vi "Set Gate Function.vi"(6 "EF":u32(ring) items=["Normal"=0, "EF_OR"=1048576, "EF_AND"=2097152, "EF_XOR"=3145728], 8 "error in (no error)":errorcluster, 9 "CD":u32(ring) items=["Normal"=0, "CD_OR"=262144, "CD_AND"=524288, "CD_XOR"=786432], 10 "AB":u32(ring) items=["Normal"=0, "AB_OR"=65536, "AB_AND"=131072, "AB_XOR"=196608], 11 "DG Number":i32) -> (0 "error out":errorcluster)   [LabVIEW 2009]
doc: "long Set_ClockParameters(BOOL ClockEnable, unsigned long DivideBy, unsigned long ClockSource, long DG_Number);"
uses:
  BME DLL/DelayGenerator.dll
panel:
  out "Result":u32 format="%08x"
  # "NOTICE -- YOU MUST LEAVE THIS NOTICE IN PLACE.  PER THE TERMS OF THE LICENSE BELOW, YOU MAY SUBLICENSE THIS SOFTWARE \nIN ANY WAY THAT DOES NOT CONFLICT WITH THIS LICENSE.\n\n### BSD License (http://www.opensource.org/licenses/bsd-license.php) Begin ###\n \nCopyright (c) 2011, Applied Energetics, http://www.appliedenergetics.com,\n                               Richard Schwerdtfeger, <rschwerdtfeger@appliedenergetics.com>\n\nAll rights reserved.\n\nRedistribution and use in source and binary forms, with or without modification, are permitted provided that the \nfollowing conditions are met:\n\n    * Redistributions of source code must retain the above copyright notice, this list of conditions and the following disclaimer.\n    * Redistributions in binary form must reproduce the above copyright notice, this list of conditions and the following disclaimer \n       in the documentation and/or other materials provided with the distribution.\n    * Neither the name of Richard Schwerdtfeger, Applied Energetics, Inc., nor the names of its contributors may be used to \n       endorse or promote products derived from this software without specific prior written permission.\n\nTHIS SOFTWARE IS PROVIDED BY THE COPYRIGHT HOLDERS AND CONTRIBUTORS \"AS IS\" AND ANY EXPRESS OR IMPLIED WARRANTIES, \nINCLUDING, BUT NOT LIMITED TO, THE IMPLIED WARRANTIES OF MERCHANTABILITY AND FITNESS FOR A PARTICULAR PURPOSE ARE \nDISCLAIMED. IN NO EVENT SHALL THE COPYRIGHT OWNER OR CONTRIBUTORS BE LIABLE FOR ANY DIRECT, INDIRECT, INCIDENTAL,\n SPECIAL, EXEMPLARY, OR CONSEQUENTIAL DAMAGES (INCLUDING, BUT NOT LIMITED TO, PROCUREMENT OF SUBSTITUTE GOODS OR \nSERVICES; LOSS OF USE, DATA, OR PROFITS; OR BUSINESS INTERRUPTION) HOWEVER CAUSED AND ON ANY THEORY OF LIABILITY, \nWHETHER IN CONTRACT, STRICT LIABILITY, OR TORT (INCLUDING NEGLIGENCE OR OTHERWISE) ARISING IN ANY WAY OUT OF THE USE \nOF THIS SOFTWARE, EVEN IF ADVISED OF THE POSSIBILITY OF SUCH DAMAGE.\n\n### BSD License End ###"
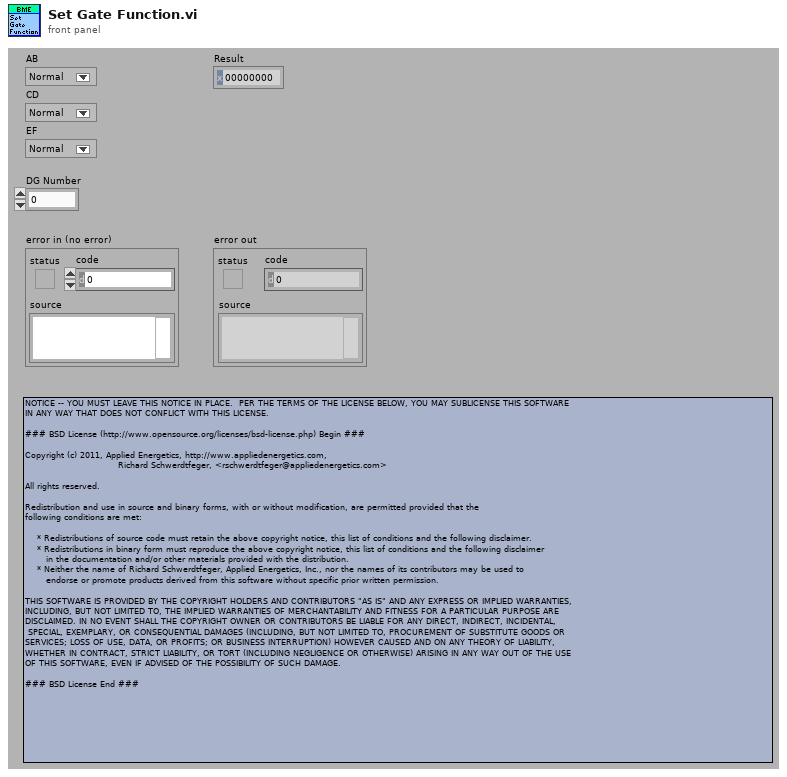
[diagram p1: front panel]
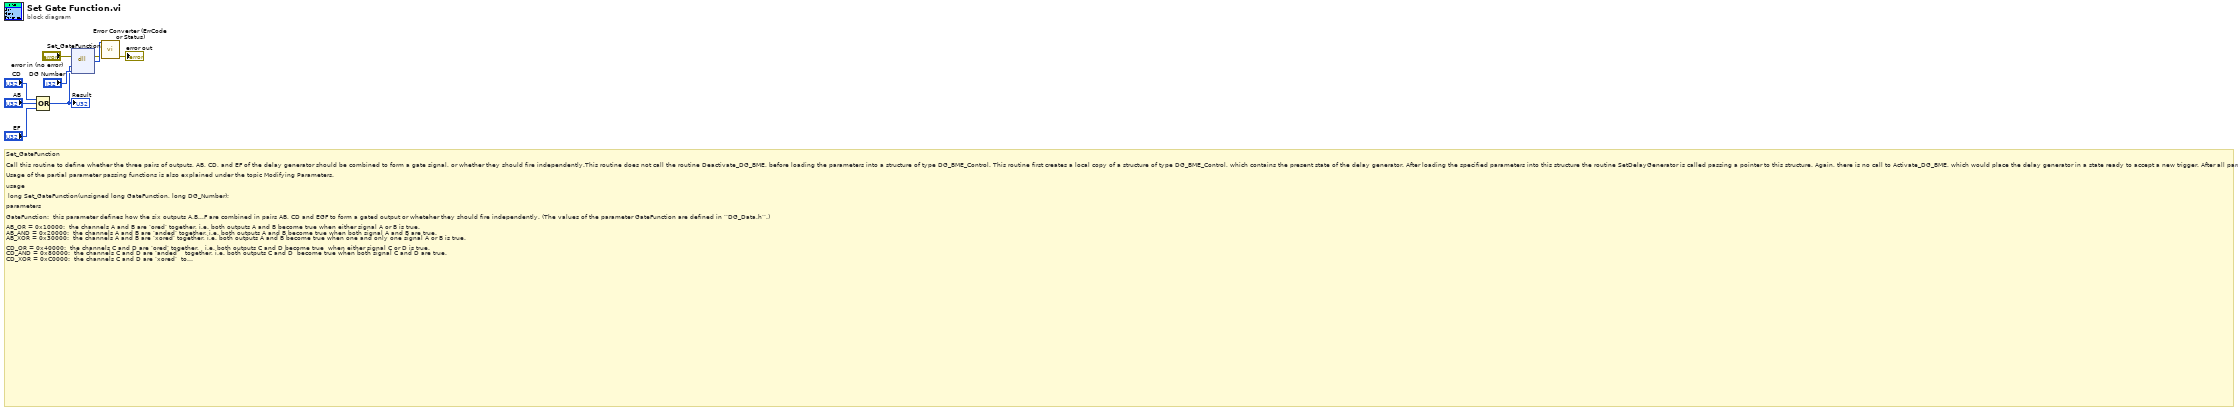
[diagram p0: block diagram]
diagram:
  # "Set_GateFunction\n\nCall this routine to define whether the three pairs of outputs, AB, CD, and EF of the delay generator should be combined to form a gate signal, or whether they should fire independently.This routine does not call the routine Deactivate_DG_BME, before loading the parameters into a structure of type DG_BME_Control. This routine first creates a local copy of a structure of type DG_BME_Control, which contains the present state of the delay generator. After loading the specified parameters into this structure the routine SetDelayGenerator is called passing a pointer to this structure. Again, there is no call to Activate_DG_BME, which would place the delay generator in a state ready to accept a new trigger. After all parameters have been loaded, an explicit call to Activate_DG_BME is necessary.\n\nUsage of the partial parameter passing functions is also explained under the topic Modifying Parameters.\n\nusage\n\n\tlong Set_GateFunction(unsigned long GateFunction, long DG_Number);\n\nparameters\n\nGateFunction:\t\tthis parameter defines how the six outputs A,B...F are combined in pairs AB, CD and EGF to form a gated output or wheteher they should fire independently. (The values of the parameter GateFunction are defined in ‘’DG_Data.h’’.)\n\nAB_OR = 0x10000:\t\tthe channels A and B are ‘ored’ together, i.e. both outputs A and B become true when either signal A or B is true.\nAB_AND = 0x20000:\t\tthe channels A and B are ‘anded’ together, i.e. both outputs A and B become true when both signal A and B are true.\nAB_XOR = 0x30000:\t\tthe channels A and B are ‘xored’ together, i.e. both outputs A and B become true when one and only one signal A or B is true.\n\nCD_OR = 0x40000:\t\tthe channels C and D are ‘ored’ together,   i.e. both outputs C and D become true  when either signal C or D is true.\nCD_AND = 0x80000:\t\tthe channels C and D are ‘anded’   together, i.e. both outputs C and D  become true when both signal C and D are true.\nCD_XOR = 0xC0000:\t\tthe channels C and D are ‘xored’  together, i.e. both outputs C and D become true when one and only one signal C or D is true.\n\nEF_OR = 0x100000:\t\tthe channels E and F are ‘ored’ together,   i.e. both outputs E and F become true  when either signal E or F is true.\nEF_AND = 0x200000:\t\tthe channels E and F are ‘anded’   together, i.e. both outputs E and F  become true when both signal E and F are true.\nEF_XOR = 0x300000:\t\tthe channels E and F are ‘xored’  together, i.e. both outputs E and F become true when one and only one signal E or F is true.\n\nDG_Number:\t\tThe number of the delay generator as assigned by the\n\nInitialize_DG_BME routine\n\nreturn value\n\n\t0:  success\n\t2:  DG_Number is out of range"
  n1 = Compound Arithmetic op=OR("CD", "AB", "EF") -> (w1:u32)
  "Result" <- w1
  n2 = dll-call lib="C:/Dokumente und Einstellungen/A2.5/Desktop/POLARIS BME DG/BME DLL/DelayGenerator.dll" fn="Set_GateFunction"(error in="error in (no error)", "Set_GateFunction"=w1, "DG_Number"="DG Number") -> (error out=w6:errorcluster, "return type"=w9:i32)  [unwired: 4 in, 1 out]
  n3 = call "Error Converter (ErrCode or Status).vi"("error in (no error)"=w6, "error code"=w9) -> ("error out"=→"error out":errorcluster)  [unwired: 9 out]
